vi "Get Gif Header.vi"(8 "error in (no error)":errorcluster caption="错误输入（无错误）", 11 "Gif Image 输入":refnum<class "Gif Image.lvclass"> caption="DNL_LabVIEW Object in") -> (0 "error out":errorcluster caption="错误输出", 1 "Version":string, 2 "Signature":string, 3 "Gif Image 输出":refnum<class "Gif Image.lvclass"> caption="DNL_LabVIEW Object out")   [LabVIEW 2012, in "Picture Box Tools.lvlib" / "Gif Image.lvclass"]
uses:
  Gif Image.lvclass
  Gif Image.lvclass/Gif Image.ctl
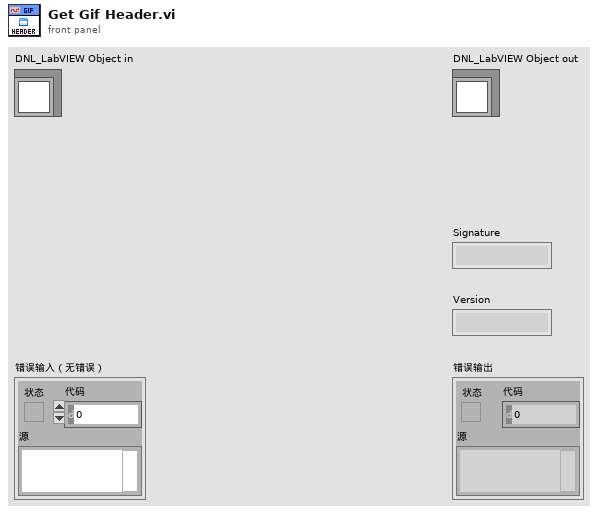
[diagram p1: front panel]
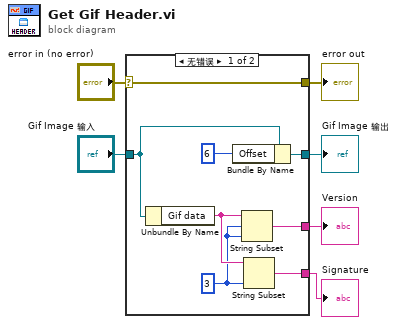
[diagram p0: block diagram]
diagram:
  n1 = case shown="无错误" "error in (no error)" {
    selector: "error in (no error)" -> [w14 w16]
    tunnel: [w14 w16] -> w5
    tunnel: [w8 w15] -> w3
    tunnel: "Gif Image 输入" -> [w9 w15]
    tunnel: [w11 _] -> w2
    tunnel: [w10 _] -> w1
    frame No Error {
      w12 = 3 ("长度（剩余）")
      n2 = Unbundle By Name(w9) -> ("Gif data"=w13:string)
      n3 = Bundle By Name(cluster=w9, "Offset"=6) -> (w8:refnum<class "Gif Image.lvclass">)
      n4 = String Subset(string=w13, offset (0)=w12, length (rest)=w12) -> (substring=w10:string)
      n5 = String Subset(string=w13, length (rest)=w12) -> (substring=w11:string)  [unwired: 1 in]
    }
    frame Error {
    }
  }
  "error out" <- w5
  "Gif Image 输出" <- w3
  "Signature" <- w2
  "Version" <- w1
